vi "Add.vi"(10 "y":dbl, 11 "x":dbl) -> (2 "x+y":dbl)   [LabVIEW 2021]
panel:
  out "Intensity Chart":dbl[][](graph)
  in  "Radio Buttons":enum32{"Radio Selection 1", "Radio Selection 2"}(radio)
  out "Boolean 3":bool
  out "Boolean 2":bool
  out "Boolean":bool
  # "MORE CHANGES MORE CHANGES"
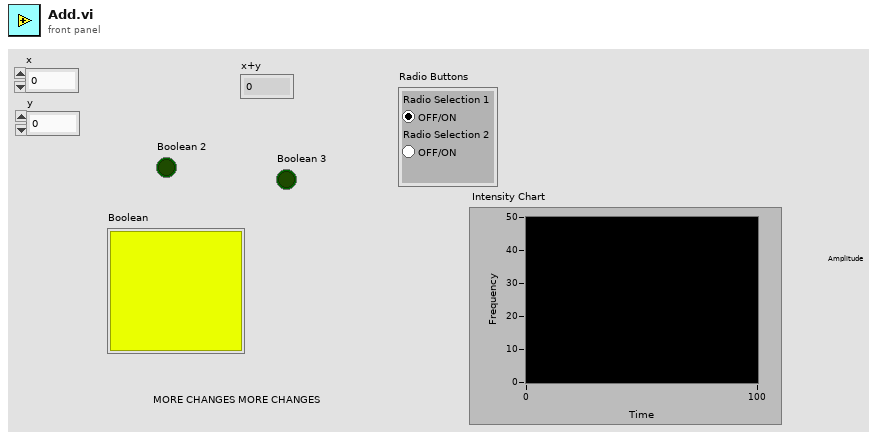
[diagram p1: front panel]
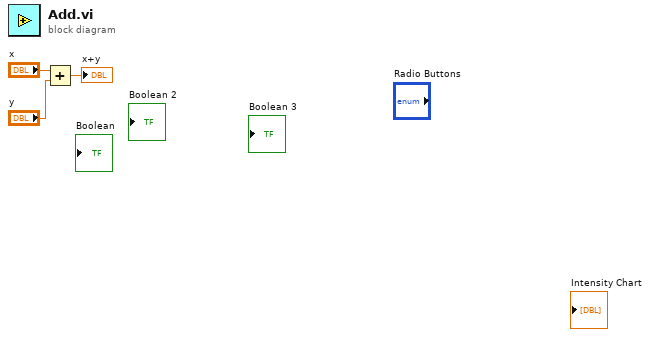
[diagram p0: block diagram]
diagram:
  n1 = Add(x="x", y="y") -> (x+y=→"x+y":dbl)
